vi "TIO Data Stream.vi"(1 "Raw Data":T3={"dstream ID"=0, "Sample Number"=417475, "Raw Data"=":-É%a\u0000J1\n\u0000É†Eï>tn\u0013Áõ9FÀó\u0010Ÿ<wm\u0010<u;Î;"}, 2 "Type(T:GMR)":bool, 3 "TIO State GMR":T1={"Awaiting REP"=FALSE, "REQ ID"=500, "dstreams in"=[], "pstreams"=[], "timebases"=[]}) -> (0 "Data Out":T2(array[cluster])=[{"Name"="gmr", "Waveform"={"start"=0.0, "dt"=1.0, "Timeseries"=[[-1045203.625, 2103369.25, -524451.0625]]}}, {"Name"="accel", "Waveform"={"start"=0.0, "dt"=1.0, "Timeseries"=[[0.4673272967338562, -9.214466094970703, -3.09728741645813]]}}, {"Name"="gyro", "Waveform"={"start"=0.0, "dt"=1.0, "Timeseries"=[[0.019417261704802513, 0.00881516095250845, 0.006293708924204111]]}}, {"Name"="bar", "Waveform"={"start"=0.0, "dt"=1.0, "Timeseries"=[[0.0]]}}, {"Name"="therm", "Waveform"={"start"=0.0, "dt"=1.0, "Timeseries"=[[0.0]]}}])   [LabVIEW 2019]
panel:
  in  "TIO State AVM":T1={"Awaiting REP"=FALSE, "REQ ID"=500, "dstreams in"=[{"id"=0, "timebase id"=1, "period"=2, "offset"=0, "sample number"=0, "total components"=3, "flags"=1, "components"=[{"pstream id"=0, "flags"=0, "period"=1, "offset"=0}, {"pstream id"=1, "flags"=0, "period"=1, "offset"=0}, {"pstream id"=2, "flags"=1, "period"=1, "offset"=0}]}, {"id"=0, "timebase id"=0, "period"=0, "offset"=0, "sample number"=0, "total components"=0, "flags"=0, "components"=[]}, {"id"=0, "timebase id"=0, "period"=0, "offset"=0, "sample number"=0, "total components"=0, "flags"=0, "components"=[]}, {"id"=0, "timebase id"=0, "period"=0, "offset"=0, "sample number"=0, "total components"=0, "flags"=0, "components"=[]}, {"id"=0, "timebase id"=0, "period"=0, "offset"=0, "sample number"=0, "total components"=0, "flags"=0, "components"=[]}, {"id"=0, "timebase id"=0, "period"=0, "offset"=0, "sample number"=0, "total components"=0, "flags"=0, "components"=[]}, {"id"=0, "timebase id"=0, "period"=0, "offset"=0, "sample number"=0, "total components"=0, "flags"=0, "components"=[]}, {"id"=0, "timebase id"=0, "period"=0, "offset"=0, "sample number"=0, "total components"=0, "flags"=0, "components"=[]}, {"id"=0, "timebase id"=0, "period"=0, "offset"=0, "sample number"=0, "total components"=0, "flags"=0, "components"=[]}, {"id"=0, "timebase id"=0, "period"=0, "offset"=0, "sample number"=0, "total components"=0, "flags"=0, "components"=[]}, {"id"=0, "timebase id"=0, "period"=0, "offset"=0, "sample number"=0, "total components"=0, "flags"=0, "components"=[]}, {"id"=0, "timebase id"=0, "period"=0, "offset"=0, "sample number"=0, "total components"=0, "flags"=0, "components"=[]}, {"id"=0, "timebase id"=0, "period"=0, "offset"=0, "sample number"=0, "total components"=0, "flags"=0, "components"=[]}, {"id"=0, "timebase id"=0, "period"=0, "offset"=0, "sample number"=0, "total components"=0, "flags"=0, "components"=[]}, {"id"=0, "timebase id"=0, "period"=0, "offset"=0, "sample number"=0, "total components"=0, "flags"=0, "components"=[]}, {"id"=0, "timebase id"=0, "period"=0, "offset"=0, "sample number"=0, "total components"=0, "flags"=0, "components"=[]}, {"id"=0, "timebase id"=0, "period"=0, "offset"=0, "sample number"=0, "total components"=0, "flags"=0, "components"=[]}, {"id"=0, "timebase id"=0, "period"=0, "offset"=0, "sample number"=0, "total components"=0, "flags"=0, "components"=[]}, {"id"=0, "timebase id"=0, "period"=0, "offset"=0, "sample number"=0, "total components"=0, "flags"=0, "components"=[]}, {"id"=0, "timebase id"=0, "period"=0, "offset"=0, "sample number"=0, "total components"=0, "flags"=0, "components"=[]}, {"id"=0, "timebase id"=0, "period"=0, "offset"=0, "sample number"=0, "total components"=0, "flags"=0, "components"=[]}, {"id"=0, "timebase id"=0, "period"=0, "offset"=0, "sample number"=0, "total components"=0, "flags"=0, "components"=[]}, {"id"=0, "timebase id"=0, "period"=0, "offset"=0, "sample number"=0, "total components"=0, "flags"=0, "components"=[]}, {"id"=0, "timebase id"=0, "period"=0, "offset"=0, "sample number"=0, "total components"=0, "flags"=0, "components"=[]}, {"id"=0, "timebase id"=0, "period"=0, "offset"=0, "sample number"=0, "total components"=0, "flags"=0, "components"=[]}, {"id"=0, "timebase id"=0, "period"=0, "offset"=0, "sample number"=0, "total components"=0, "flags"=0, "components"=[]}, {"id"=0, "timebase id"=0, "period"=0, "offset"=0, "sample number"=0, "total components"=0, "flags"=0, "components"=[]}, {"id"=0, "timebase id"=0, "period"=0, "offset"=0, "sample number"=0, "total components"=0, "flags"=0, "components"=[]}, {"id"=0, "timebase id"=0, "period"=0, "offset"=0, "sample number"=0, "total components"=0, "flags"=0, "components"=[]}, {"id"=0, "timebase id"=0, "period"=0, "offset"=0, "sample number"=0, "total components"=0, "flags"=0, "components"=[]}, {"id"=0, "timebase id"=0, "period"=0, "offset"=0, "sample number"=0, "total components"=0, "flags"=0, "components"=[]}, {"id"=0, "timebase id"=0, "period"=0, "offset"=0, "sample number"=0, "total components"=0, "flags"=0, "components"=[]}], "pstreams"=[{"id"=0, "timebase_id"=1, "period"=1, "offset"=0, "fmt"=-1, "flags"=0, "channels"=1, "type"=130, "name"="avm", "column names"=["x"], "title"="Field", "units"="nT"}, {"id"=1, "timebase_id"=1, "period"=1, "offset"=0, "fmt"=-1, "flags"=0, "channels"=1, "type"=16, "name"="signal", "column names"=["x"], "title"="Signal", "units"="NA"}, {"id"=2, "timebase_id"=1, "period"=8, "offset"=0, "fmt"=-1, "flags"=0, "channels"=1, "type"=16, "name"="Stat", "column names"=["Stat"], "title"="Status", "units"="NA"}, {"id"=3, "timebase_id"=1, "period"=80, "offset"=0, "fmt"=-1, "flags"=0, "channels"=1, "type"=66, "name"="bar", "column names"=[""], "title"="Atmospheric pressure", "units"="mbar"}, {"id"=4, "timebase_id"=1, "period"=80, "offset"=0, "fmt"=-1, "flags"=0, "channels"=1, "type"=66, "name"="therm", "column names"=[""], "title"="Ambient temperature", "units"="C"}, {"id"=0, "timebase_id"=0, "period"=0, "offset"=0, "fmt"=0, "flags"=0, "channels"=0, "type"=0, "name"="", "column names"=[], "title"="", "units"=""}, {"id"=0, "timebase_id"=0, "period"=0, "offset"=0, "fmt"=0, "flags"=0, "channels"=0, "type"=0, "name"="", "column names"=[], "title"="", "units"=""}, {"id"=0, "timebase_id"=0, "period"=0, "offset"=0, "fmt"=0, "flags"=0, "channels"=0, "type"=0, "name"="", "column names"=[], "title"="", "units"=""}, {"id"=0, "timebase_id"=0, "period"=0, "offset"=0, "fmt"=0, "flags"=0, "channels"=0, "type"=0, "name"="", "column names"=[], "title"="", "units"=""}, {"id"=0, "timebase_id"=0, "period"=0, "offset"=0, "fmt"=0, "flags"=0, "channels"=0, "type"=0, "name"="", "column names"=[], "title"="", "units"=""}, {"id"=0, "timebase_id"=0, "period"=0, "offset"=0, "fmt"=0, "flags"=0, "channels"=0, "type"=0, "name"="", "column names"=[], "title"="", "units"=""}, {"id"=0, "timebase_id"=0, "period"=0, "offset"=0, "fmt"=0, "flags"=0, "channels"=0, "type"=0, "name"="", "column names"=[], "title"="", "units"=""}, {"id"=0, "timebase_id"=0, "period"=0, "offset"=0, "fmt"=0, "flags"=0, "channels"=0, "type"=0, "name"="", "column names"=[], "title"="", "units"=""}, {"id"=0, "timebase_id"=0, "period"=0, "offset"=0, "fmt"=0, "flags"=0, "channels"=0, "type"=0, "name"="", "column names"=[], "title"="", "units"=""}, {"id"=0, "timebase_id"=0, "period"=0, "offset"=0, "fmt"=0, "flags"=0, "channels"=0, "type"=0, "name"="", "column names"=[], "title"="", "units"=""}, {"id"=0, "timebase_id"=0, "period"=0, "offset"=0, "fmt"=0, "flags"=0, "channels"=0, "type"=0, "name"="", "column names"=[], "title"="", "units"=""}, {"id"=32768, "timebase_id"=1, "period"=1, "offset"=0, "fmt"=-1, "flags"=0, "channels"=3, "type"=66, "name"="_gmr.raw", "column names"=["x", "y", "z"], "title"="Vector magnetic field", "units"="nT"}, {"id"=32769, "timebase_id"=1, "period"=8, "offset"=0, "fmt"=-1, "flags"=0, "channels"=3, "type"=66, "name"="_accel.raw", "column names"=["x", "y", "z"], "title"="Acceleration", "units"="m/s^2"}, {"id"=32770, "timebase_id"=1, "period"=8, "offset"=0, "fmt"=-1, "flags"=0, "channels"=3, "type"=66, "name"="_gyro.raw", "column names"=["x", "y", "z"], "title"="Angular velocity", "units"="rad/s"}, {"id"=32771, "timebase_id"=1, "period"=80, "offset"=0, "fmt"=-1, "flags"=0, "channels"=1, "type"=66, "name"="_bar.raw", "column names"=[""], "title"="Atmospheric pressure", "units"="mbar"}, {"id"=32772, "timebase_id"=1, "period"=80, "offset"=0, "fmt"=-1, "flags"=0, "channels"=1, "type"=66, "name"="_therm.raw", "column names"=[""], "title"="Ambient temperature", "units"="C"}, {"id"=32773, "timebase_id"=0, "period"=1, "offset"=0, "fmt"=-1, "flags"=0, "channels"=1, "type"=66, "name"="_cpu.raw", "column names"=[""], "title"="CPU load", "units"="%"}, {"id"=32774, "timebase_id"=0, "period"=1, "offset"=0, "fmt"=-1, "flags"=0, "channels"=1, "type"=66, "name"="cpu", "column names"=[""], "title"="CPU load", "units"="%"}, {"id"=0, "timebase_id"=0, "period"=0, "offset"=0, "fmt"=0, "flags"=0, "channels"=0, "type"=0, "name"="", "column names"=[], "title"="", "units"=""}, {"id"=0, "timebase_id"=0, "period"=0, "offset"=0, "fmt"=0, "flags"=0, "channels"=0, "type"=0, "name"="", "column names"=[], "title"="", "units"=""}, {"id"=0, "timebase_id"=0, "period"=0, "offset"=0, "fmt"=0, "flags"=0, "channels"=0, "type"=0, "name"="", "column names"=[], "title"="", "units"=""}, {"id"=0, "timebase_id"=0, "period"=0, "offset"=0, "fmt"=0, "flags"=0, "channels"=0, "type"=0, "name"="", "column names"=[], "title"="", "units"=""}, {"id"=0, "timebase_id"=0, "period"=0, "offset"=0, "fmt"=0, "flags"=0, "channels"=0, "type"=0, "name"="", "column names"=[], "title"="", "units"=""}, {"id"=0, "timebase_id"=0, "period"=0, "offset"=0, "fmt"=0, "flags"=0, "channels"=0, "type"=0, "name"="", "column names"=[], "title"="", "units"=""}, {"id"=0, "timebase_id"=0, "period"=0, "offset"=0, "fmt"=0, "flags"=0, "channels"=0, "type"=0, "name"="", "column names"=[], "title"="", "units"=""}, {"id"=0, "timebase_id"=0, "period"=0, "offset"=0, "fmt"=0, "flags"=0, "channels"=0, "type"=0, "name"="", "column names"=[], "title"="", "units"=""}, {"id"=0, "timebase_id"=0, "period"=0, "offset"=0, "fmt"=0, "flags"=0, "channels"=0, "type"=0, "name"="", "column names"=[], "title"="", "units"=""}], "timebases"=[{"id"=0, "source"=1, "epoch"=0, "start time"=0, "period numerator (µs)"=100000000, "period denominator (µs)"=1000, "flags"=0, "stability"=1.0, "source id"="\u0000\u0000\u0000¬Å'7\u0001\u0000\u0000\u0000B\u0000!\u0000\u0011P6W462 "}, {"id"=1, "source"=1, "epoch"=248, "start time"=0, "period numerator (µs)"=1250000, "period denominator (µs)"=1000, "flags"=0, "stability"=1.0, "source id"="\u0000\u0000\u0000¬Å'7\u0001\u0000\u0000\u0000B\u0000!\u0000\u0011P6W462 "}, {"id"=0, "source"=0, "epoch"=0, "start time"=0, "period numerator (µs)"=0, "period denominator (µs)"=0, "flags"=0, "stability"=0.0, "source id"=""}, {"id"=0, "source"=0, "epoch"=0, "start time"=0, "period numerator (µs)"=0, "period denominator (µs)"=0, "flags"=0, "stability"=0.0, "source id"=""}, {"id"=0, "source"=0, "epoch"=0, "start time"=0, "period numerator (µs)"=0, "period denominator (µs)"=0, "flags"=0, "stability"=0.0, "source id"=""}, {"id"=0, "source"=0, "epoch"=0, "start time"=0, "period numerator (µs)"=0, "period denominator (µs)"=0, "flags"=0, "stability"=0.0, "source id"=""}, {"id"=0, "source"=0, "epoch"=0, "start time"=0, "period numerator (µs)"=0, "period denominator (µs)"=0, "flags"=0, "stability"=0.0, "source id"=""}, {"id"=0, "source"=0, "epoch"=0, "start time"=0, "period numerator (µs)"=0, "period denominator (µs)"=0, "flags"=0, "stability"=0.0, "source id"=""}, {"id"=0, "source"=0, "epoch"=0, "start time"=0, "period numerator (µs)"=0, "period denominator (µs)"=0, "flags"=0, "stability"=0.0, "source id"=""}, {"id"=0, "source"=0, "epoch"=0, "start time"=0, "period numerator (µs)"=0, "period denominator (µs)"=0, "flags"=0, "stability"=0.0, "source id"=""}, {"id"=0, "source"=0, "epoch"=0, "start time"=0, "period numerator (µs)"=0, "period denominator (µs)"=0, "flags"=0, "stability"=0.0, "source id"=""}, {"id"=0, "source"=0, "epoch"=0, "start time"=0, "period numerator (µs)"=0, "period denominator (µs)"=0, "flags"=0, "stability"=0.0, "source id"=""}, {"id"=0, "source"=0, "epoch"=0, "start time"=0, "period numerator (µs)"=0, "period denominator (µs)"=0, "flags"=0, "stability"=0.0, "source id"=""}, {"id"=0, "source"=0, "epoch"=0, "start time"=0, "period numerator (µs)"=0, "period denominator (µs)"=0, "flags"=0, "stability"=0.0, "source id"=""}, {"id"=0, "source"=0, "epoch"=0, "start time"=0, "period numerator (µs)"=0, "period denominator (µs)"=0, "flags"=0, "stability"=0.0, "source id"=""}, {"id"=0, "source"=0, "epoch"=0, "start time"=0, "period numerator (µs)"=0, "period denominator (µs)"=0, "flags"=0, "stability"=0.0, "source id"=""}, {"id"=0, "source"=0, "epoch"=0, "start time"=0, "period numerator (µs)"=0, "period denominator (µs)"=0, "flags"=0, "stability"=0.0, "source id"=""}, {"id"=0, "source"=0, "epoch"=0, "start time"=0, "period numerator (µs)"=0, "period denominator (µs)"=0, "flags"=0, "stability"=0.0, "source id"=""}, {"id"=0, "source"=0, "epoch"=0, "start time"=0, "period numerator (µs)"=0, "period denominator (µs)"=0, "flags"=0, "stability"=0.0, "source id"=""}, {"id"=0, "source"=0, "epoch"=0, "start time"=0, "period numerator (µs)"=0, "period denominator (µs)"=0, "flags"=0, "stability"=0.0, "source id"=""}, {"id"=0, "source"=0, "epoch"=0, "start time"=0, "period numerator (µs)"=0, "period denominator (µs)"=0, "flags"=0, "stability"=0.0, "source id"=""}, {"id"=0, "source"=0, "epoch"=0, "start time"=0, "period numerator (µs)"=0, "period denominator (µs)"=0, "flags"=0, "stability"=0.0, "source id"=""}, {"id"=0, "source"=0, "epoch"=0, "start time"=0, "period numerator (µs)"=0, "period denominator (µs)"=0, "flags"=0, "stability"=0.0, "source id"=""}, {"id"=0, "source"=0, "epoch"=0, "start time"=0, "period numerator (µs)"=0, "period denominator (µs)"=0, "flags"=0, "stability"=0.0, "source id"=""}, {"id"=0, "source"=0, "epoch"=0, "start time"=0, "period numerator (µs)"=0, "period denominator (µs)"=0, "flags"=0, "stability"=0.0, "source id"=""}, {"id"=0, "source"=0, "epoch"=0, "start time"=0, "period numerator (µs)"=0, "period denominator (µs)"=0, "flags"=0, "stability"=0.0, "source id"=""}, {"id"=0, "source"=0, "epoch"=0, "start time"=0, "period numerator (µs)"=0, "period denominator (µs)"=0, "flags"=0, "stability"=0.0, "source id"=""}, {"id"=0, "source"=0, "epoch"=0, "start time"=0, "period numerator (µs)"=0, "period denominator (µs)"=0, "flags"=0, "stability"=0.0, "source id"=""}, {"id"=0, "source"=0, "epoch"=0, "start time"=0, "period numerator (µs)"=0, "period denominator (µs)"=0, "flags"=0, "stability"=0.0, "source id"=""}, {"id"=0, "source"=0, "epoch"=0, "start time"=0, "period numerator (µs)"=0, "period denominator (µs)"=0, "flags"=0, "stability"=0.0, "source id"=""}, {"id"=0, "source"=0, "epoch"=0, "start time"=0, "period numerator (µs)"=0, "period denominator (µs)"=0, "flags"=0, "stability"=0.0, "source id"=""}, {"id"=0, "source"=0, "epoch"=0, "start time"=0, "period numerator (µs)"=0, "period denominator (µs)"=0, "flags"=0, "stability"=0.0, "source id"=""}]}
  # "TIO Data Stream Process"
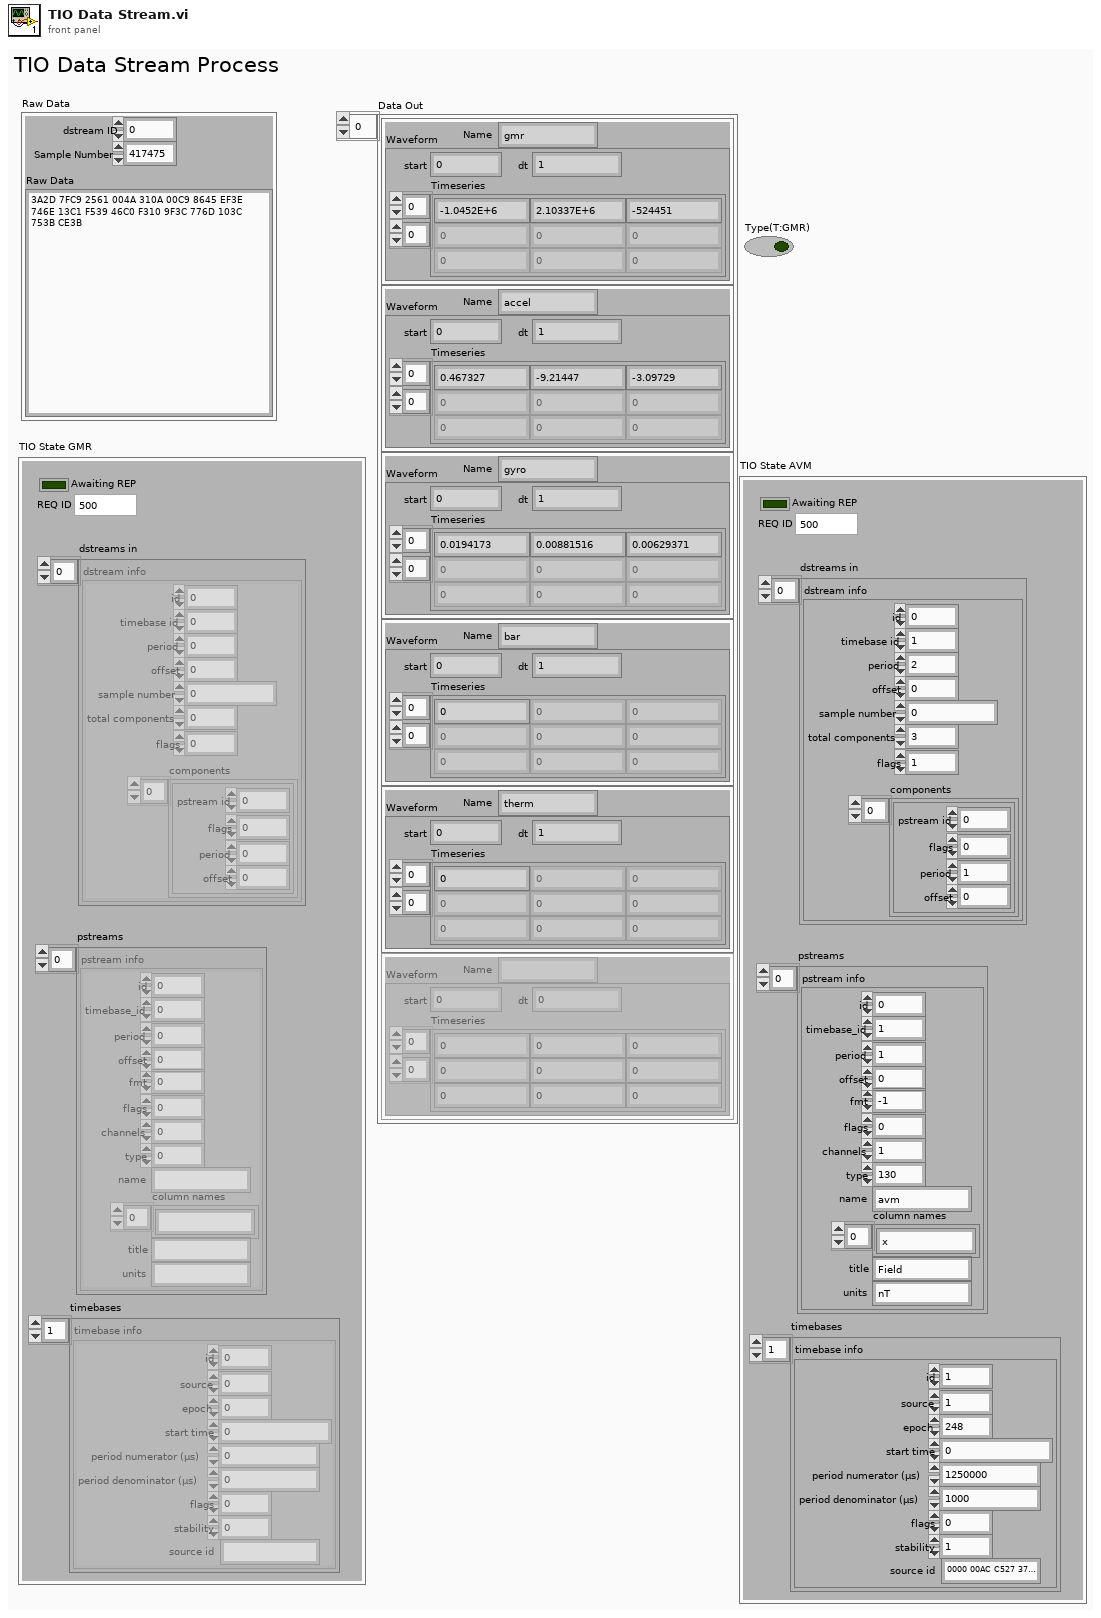
[diagram p1: front panel]
types:
  T1 = cluster{"Awaiting REP":bool, "REQ ID":u32, "dstreams in":cluster{"id":u16, "timebase id":u16, "period":u32, "offset":u32, "sample number":u64, "total components":u16, "flags":u16, "components":cluster{"pstream id":u16, "flags":u16, "period":u32, "offset":u32}[]}[], "pstreams":cluster{"id":u16, "timebase_id":u16, "period":u32, "offset":u32, "fmt":i32, "flags":u16, "channels":u16, "type":u8, "name":string, "column names":string[], "title":string, "units":string}[], "timebases":cluster{"id":u16, "source":u8, "epoch":u8, "start time":u64, "period numerator (µs)":u32, "period denominator (µs)":u32, "flags":u32, "stability":sgl, "source id":string}[]}
  T2 = cluster{"Name":string, "Waveform":cluster{"start":dbl, "dt":dbl, "Timeseries":dbl[][]}}[]
  T3 = cluster{"dstream ID":u16, "Sample Number":u32, "Raw Data":string}
  T4 = cluster{"id":u16, "source":u8, "epoch":u8, "start time":u64, "period numerator (µs)":u32, "period denominator (µs)":u32, "flags":u32, "stability":sgl, "source id":string}[]
  T5 = cluster{"id":u16, "timebase_id":u16, "period":u32, "offset":u32, "fmt":i32, "flags":u16, "channels":u16, "type":u8, "name":string, "column names":string[], "title":string, "units":string}[]
  T6 = cluster{"id":u16, "timebase id":u16, "period":u32, "offset":u32, "sample number":u64, "total components":u16, "flags":u16, "components":cluster{"pstream id":u16, "flags":u16, "period":u32, "offset":u32}[]}[]
  T7 = cluster{"id":u16, "timebase id":u16, "period":u32, "offset":u32, "sample number":u64, "total components":u16, "flags":u16, "components":cluster{"pstream id":u16, "flags":u16, "period":u32, "offset":u32}[]}
  T8 = cluster{"pstream id":u16, "flags":u16, "period":u32, "offset":u32}[]
  T9 = cluster{"id":u16, "source":u8, "epoch":u8, "start time":u64, "period numerator (µs)":u32, "period denominator (µs)":u32, "flags":u32, "stability":sgl, "source id":string}
  T10 = enum16{"big-endian, network order", "native, host order", "little-endian"}
  T11 = cluster{"id":u16, "timebase_id":u16, "period":u32, "offset":u32, "fmt":i32, "flags":u16, "channels":u16, "type":u8, "name":string, "column names":string[], "title":string, "units":string}
  T12 = cluster{"name":string, cluster{dbl, dbl, dbl[][]}}
  T13 = cluster{"name":string, cluster{dbl, dbl, dbl[][]}}[]
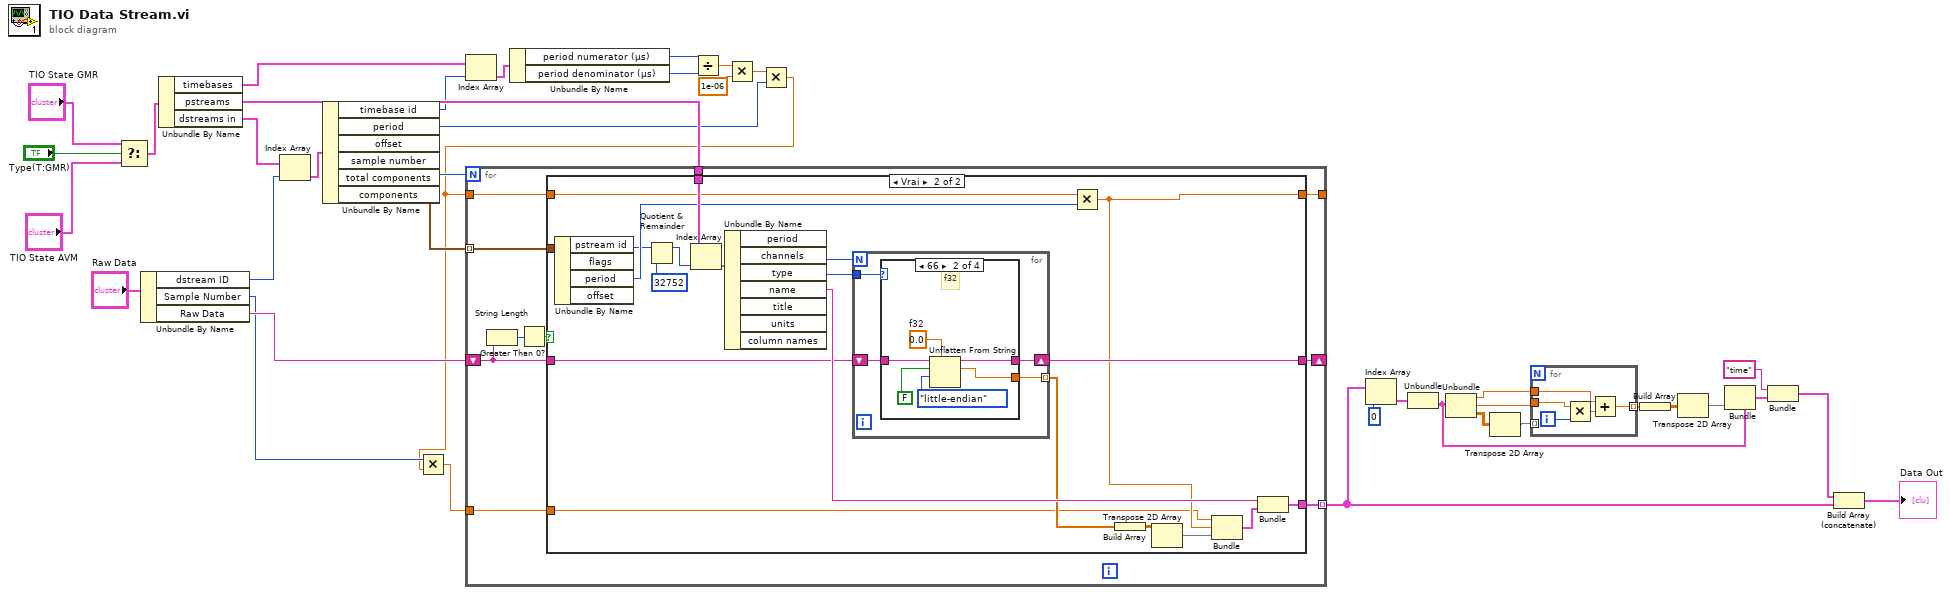
[diagram p0: block diagram]
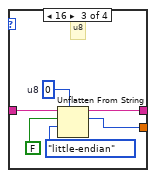
[diagram p4: hidden frame]
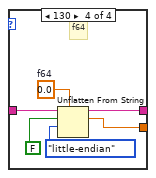
[diagram p5: hidden frame]
diagram:
  n1 = Select(t="TIO State GMR", s="Type(T:GMR)", f="TIO State AVM") -> (s? t:f=w2:T1)
  n2 = Unbundle By Name("Raw Data") -> ("dstream ID"=w38:u16, "Sample Number"=w7:u32, "Raw Data"=w32:string)
  n3 = Unbundle By Name(w2) -> ("timebases"=w30:T4, "pstreams"=w33:T5, "dstreams in"=w37:T6)
  n4 = Index Array(array=w37, index=w38) -> (element=w36:T7)
  n5 = Unbundle By Name(w36) -> ("timebase id"=w31:u16, "period"=w24:u32, "total components"=w35:u16, "components"=w34:T8)  [unwired: 2 out]
  n6 = Index Array(array=w30, index=w31) -> (element=w29:T9)
  n7 = Unbundle By Name(w29) -> ("period numerator (µs)"=w28:u32, "period denominator (µs)"=w27:u32)
  n8 = Divide(x=w28, y=w27) -> (x/y=w26:dbl)
  n9 = Multiply(x=w26, y=1e-06) -> (x*y=w25:dbl)
  n10 = Multiply(x=w25, y=w24) -> (x*y=w5:dbl)
  n11 = Multiply(x=w7, y=w5) -> (x*y=w6:dbl)
  n12 = for {
    N: w35 -> [_]
    tunnel: w34 -> [w49] mode=indexing
    tunnel: w33 -> [w48]
    shift-right: [w47] -> _
    shift-left: w32 -> [w45]
    tunnel: [w46] -> w21 mode=indexing
    tunnel: w6 -> [w40]
    tunnel: w5 -> [w41]
    tunnel: [w42] -> _
    n13 = String Length(string=w45) -> (length=w44:i32)
    n14 = Greater Than 0?(x=w44) -> (x > 0?=w43:bool)
    n15 = case shown="Vrai" w43 {
      tunnel: w49 -> [_ w71]
      tunnel: w48 -> [_ w70]
      tunnel: [w51 w66] -> w47
      tunnel: [_ w64] -> w46
      tunnel: w45 -> [w51 w61]
      tunnel: w41 -> [w50 w58]
      tunnel: [w50 w57] -> w42
      tunnel: w40 -> [_ w56]
      frame False {
      }
      frame True {
        n16 = Unbundle By Name(w71) -> ("pstream id"=w53:u16, "period"=w55:u32)  [unwired: 2 out]
        n17 = Quotient & Remainder(x=w53, y=u16 32752) -> (x-y*floor(x/y)=w52:u16)  [unwired: 1 out]
        n18 = Index Array(array=w70, index=w52) -> (element=w69:T11)
        n19 = Unbundle By Name(w69) -> ("channels"=w68:u16, "type"=w67:u8, "name"=w65:string)  [unwired: 4 out]
        n20 = for {
          N: w68 -> [_]
          tunnel: w67 -> [w75]
          tunnel: [w74] -> w63 mode=indexing
          shift-right: [w73] -> w66
          shift-left: w61 -> [w72]
          n21 = case shown="66" w75 {
            tunnel: w72 -> [_ w81 w87 w93]
            tunnel: [_ w77 w83 w89] -> w74
            tunnel: [_ w76 w82 w88] -> w73
            frame 0, Default {
            }
            frame 66 {
              w78 = sgl 0.0  # f32
              # "f32"
              n22 = Unflatten From String(type=w78, binary string=w81, data includes array or string size? (T)=FALSE, byte order (0:big-endian, network order)=T10."little-endian") -> (rest of the binary string=w76:string, value=w77:sgl)  [unwired: 1 in, 1 out]
            }
            frame 16 {
              w84 = u8 0  # u8
              # "u8"
              n23 = Unflatten From String(type=w84, binary string=w87, data includes array or string size? (T)=FALSE, byte order (0:big-endian, network order)=T10."little-endian") -> (rest of the binary string=w82:string, value=w83:u8)  [unwired: 1 in, 1 out]
            }
            frame 130 {
              w90 = 0.0  # f64
              # "f64"
              n24 = Unflatten From String(type=w90, binary string=w93, data includes array or string size? (T)=FALSE, byte order (0:big-endian, network order)=T10."little-endian") -> (rest of the binary string=w88:string, value=w89:dbl)  [unwired: 1 in, 1 out]
            }
          }
        }
        n25 = Multiply(x=w58, y=w55) -> (x*y=w57:dbl)
        n26 = Build Array(w63) -> (w60:dbl[][])
        n27 = Transpose 2D Array(2D array=w60) -> (transposed array=w59:dbl[][])
        n28 = Bundle(w56, w57, w59) -> (w62:cluster{dbl, dbl, dbl[][]})  [unwired: 1 in]
        n29 = Bundle("name"=w65, w62) -> (w64:T12)  [unwired: 1 in]
      }
    }
  }
  n30 = Index Array(array=w21, index=0) -> (element=w19:T12)
  n31 = Unbundle(w19) -> (w16:cluster{dbl, dbl, dbl[][]})  [unwired: 1 out]
  n32 = Unbundle(w16) -> (w17:dbl, w18:dbl, w9:dbl[][])
  n33 = Transpose 2D Array(2D array=w9) -> (transposed array=w8:dbl[][])
  n34 = for {
    tunnel: w17 -> [w95]
    tunnel: w18 -> [w97]
    tunnel: [w94] -> w13 mode=indexing
    tunnel: w8 -> [_] mode=indexing
    i -> [w98]
    n35 = Multiply(x=w97, y=w98) -> (x*y=w96:dbl)
    n36 = Add(x=w95, y=w96) -> (x+y=w94:dbl)
  }
  n37 = Build Array(w13) -> (w12:dbl[][])
  n38 = Transpose 2D Array(2D array=w12) -> (transposed array=w11:dbl[][])
  n39 = Bundle(cluster=w16, w11) -> (w15:cluster{dbl, dbl, dbl[][]})  [unwired: 2 in]
  n40 = Bundle("time", w15) -> (w10:cluster{string, cluster{dbl, dbl, dbl[][]}})  [unwired: 1 in]
  n41 = Build Array (concatenate)(w10, w21) -> (→"Data Out":T13)
